vi "RunFP.vi"(0 "VI refnum in":refnum<vi>, 5 "Wait until VI done?":bool caption="Wait until VI done? (F)", 7 "Auto dispose VI refnum?":bool=TRUE caption="Auto dispose VI refnum? (T)", 11 "Error in":errorcluster caption="Error in (no error)", 12 "Control names":string[](array[string]) caption="Control names (none)", 13 "Control values":variant[](array[variant]) caption="Control values (none)") -> (4 "VI refnum out":refnum<vi>, 6 "VI running?":bool, 8 "Last execution state":T1(ring), 14 "Control values set?":bool, 15 "Error out":errorcluster)   [LabVIEW 2017, in "VILauncher.lvlib"]
doc: "Runs the dynamic VI specified by <B>VI refnum in</B>.\n\nThis function will wait until the dynamic VI is done if <B>Wait until VI done?</B> is True (default is False), and it will auto dispose the dynamic VI reference (hand it over to the running dynamic VI) if <B>Auto dispose VI refnum?</B> is True. Note that if this function fails to run the VI, <B>VI refnum in</B> will not be auto-disposed, in which case you retain the responsibility of closing that reference yourself.\n\nThe <B>VI running?</B> output will only be True if the dynamic VI's <B>Last execution state</B> is \"Run top level\". <B>VI running?</B> can be False even if the dynamic VI ran successfully - it might just have finished before this VI finished.\n\nOptionally you can send input data to the dynamic VI when running it using one of two modes; Right click this VI and use the Select Type menu to choose input data transfer mode:\n\nInput data via front panel\n-------------------------------\nSet data on the front panel of the dynamic VI before running it by wiring <B>Control names</B> and <B>Control values</B>. <B>Control values set?</B> will be True only if all <B>Control names</B> were valid.\n\nInput data via block diagram\n----------------------------------\nTransmit data to the dynamic VI after it has started by wiring <B>Input data names</B> and <B>Input data values</B>. If you use this mode the dynamic VI must use the WaitForInputData function to read the input data on the block diagram. The read in the dynamic VI must be finished before <B>Input data timeout</B> runs out. Set this timeout value to -1 (default) to wait indefinitely. If timeout does occur, <B>Input data timed out?</B> will be True. <B>Input data delivered?</B> will be True only if input data was in fact transmitted to the dynamic VI without any errors.\n\n<B>NOTE 1:</B> When using the 'Input data via block diagram' mode the dynamic VI must use the WaitForInputData function even if you send zero input data. To avoid this requirement for the dynamic VI when not passing any input data, please use the 'Input data via front panel' mode in this case.\n\n<B>NOTE 2:</B> The dynamic VI must have its front panel available at runtime for this function to work. The simplest way to ensure this, which also works in a built application without additional steps to be taken, is by enabling \"Show front panel when called\" in the \"Window Appearance\" section of the dynamic VI Properties.\n\nThis VI is reentrant, and it will run only if there is no error on <B>Error in</B>.\n\nSteen Schmidt\nGPower\n2/1 2013"
uses:
  VILauncher.lvlib
  Error/GPError.lvlib
panel:
  # "Copyright © 2013\nGPower\nSee enclosed license file for terms and conditions"
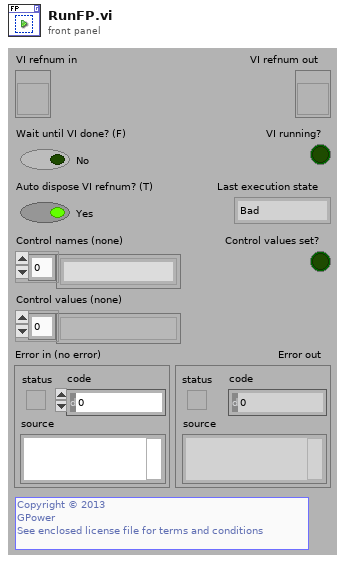
[diagram p1: front panel]
types:
  T1 = enum32{"Bad", "Idle", "Run top level", "Running"}
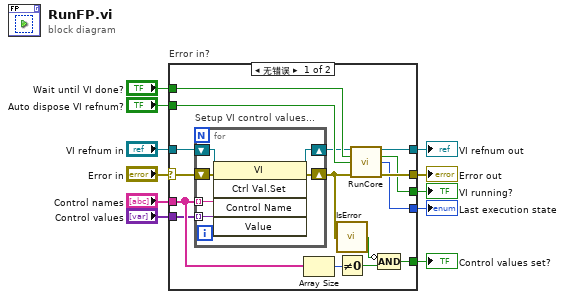
[diagram p0: block diagram]
diagram:
  n1 = case "Error in?" shown="无错误" "Error in" {
    selector: "Error in" -> [w13 w35]
    tunnel: [w25 w35] -> w10
    tunnel: "Control names" -> [w27 _]
    tunnel: "Control values" -> [w26 _]
    tunnel: [w24 w34] -> w9
    tunnel: "Auto dispose VI refnum?" -> [w23 _]
    tunnel: [w22 _] -> w7
    tunnel: [w21 _] -> w6
    tunnel: "Wait until VI done?" -> [w20 _]
    tunnel: [w19 _] -> w4
    tunnel: "VI refnum in" -> [w15 w34]
    frame No Error {
      n2 = for "Setup VI control values..." {
        shift-right: [w32] -> w12
        shift-left: w13 -> [w33]
        tunnel: w27 -> [w30] mode=indexing
        tunnel: w26 -> [w29] mode=indexing
        shift-right: [w28] -> w14
        shift-left: w15 -> [w31]
        n3 = invoke class="VI" method="Ctrl Val.Set"(reference=w31, error in=w33, "Control Name"=w30, "Value"=w29) -> (reference out=w28:refnum<vi>, error out=w32:errorcluster)  [unwired: 1 in, 3 out]
      }
      n4 = Array Size(array=w27) -> (size(s)=w18:i32)
      n5 = call "IsError.vi"("Error in"=w12) -> ("Error?"=w16:bool)  [unwired: 4 in]
      n6 = Not Equal To 0?(x=w18) -> (x != 0?=w17:bool)
      n7 = call "RunCore.vi"("VI refnum in"=w14, "Wait until VI done?"=w20, "Auto dispose VI refnum?"=w23, "Error in"=w12) -> ("VI refnum out"=w24:refnum<vi>, "VI running?"=w22:bool, "Last execution state"=w21:T1, "Error out"=w25:errorcluster)  [unwired: 8 in]
      n8 = Compound Arithmetic op=AND(invert w16, w17) -> (w19:bool)
    }
    frame Error {
    }
  }
  "Error out" <- w10
  "VI refnum out" <- w9
  "VI running?" <- w7
  "Last execution state" <- w6
  "Control values set?" <- w4
